vi "BoxcarAverage.vi"(2 "IR Sensors In":T1(array[cluster]), 3 "Box Car Average In":dbl[][](array[numeric])) -> (0 "IR Sensors Out":T1(array[cluster]), 1 "Box Car Average Out":dbl[][](array[numeric]))   [LabVIEW 2014]
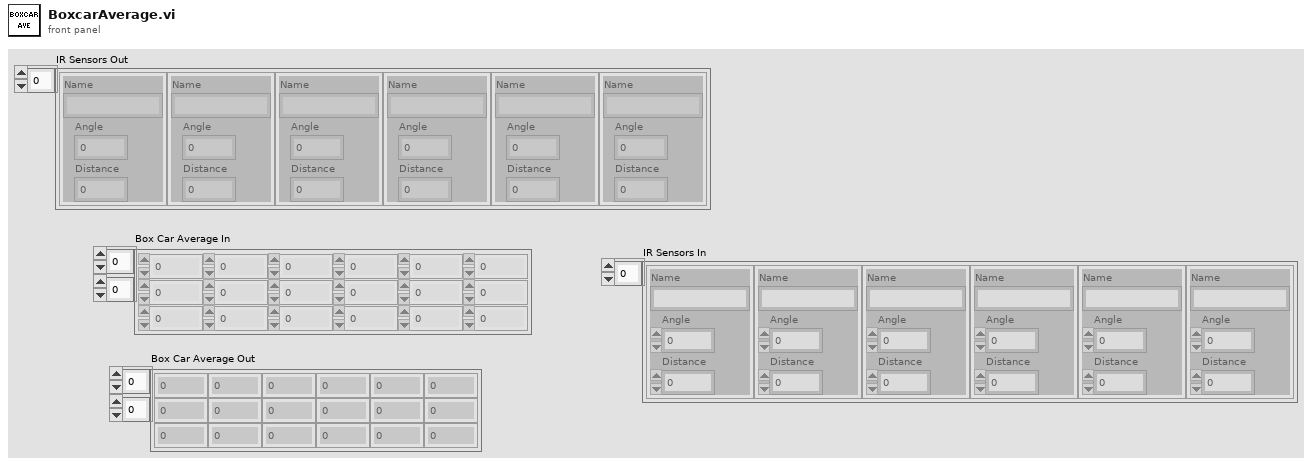
[diagram p1: front panel]
types:
  T1 = cluster{"Name":string, "Angle":dbl, "Distance":dbl}[]
  T2 = cluster{"Name":string, "Angle":dbl, "Distance":dbl}
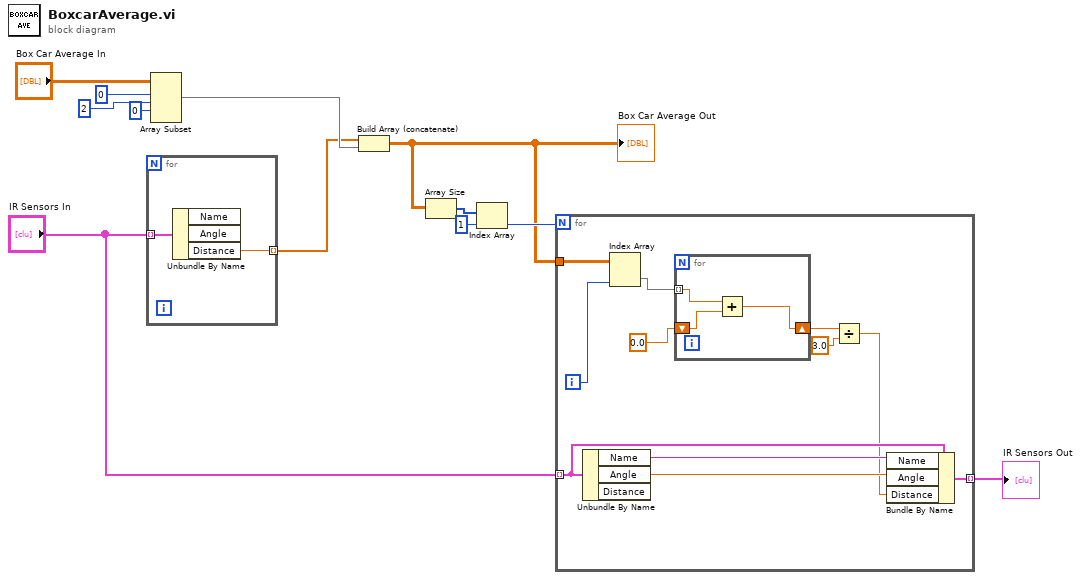
[diagram p0: block diagram]
diagram:
  n1 = for {
    tunnel: "IR Sensors In" -> [w14] mode=indexing
    tunnel: [w13] -> w7 mode=indexing
    n2 = Unbundle By Name(w14) -> ("Distance"=w13:dbl)  [unwired: 2 out]
  }
  n3 = Array Subset(array="Box Car Average In", index (row)=0 ("index"), length (row)=2 ("length"), index (col)=0 ("index")) -> (w8:dbl[][])  [unwired: 1 in]
  n4 = Build Array (concatenate)(w7, w8) -> (w3:dbl[][])
  "Box Car Average Out" <- w3
  n5 = Array Size(array=w3) -> (size(s)=w6:i32[])
  n6 = Index Array(array=w6, index=1) -> (element=w4:i32)
  n7 = for {
    N: w4 -> [_]
    tunnel: w3 -> [w25]
    tunnel: "IR Sensors In" -> [w19] mode=indexing
    tunnel: [w15] -> w1 mode=indexing
    i -> [w24]
    n8 = Unbundle By Name(w19) -> ("Name"=w18:string, "Angle"=w17:dbl)  [unwired: 1 out]
    n9 = Index Array(array=w25, index (col)=w24) -> (element=w23:dbl[])  [unwired: 1 in]
    n10 = for {
      tunnel: w23 -> [w28] mode=indexing
      shift-right: [w26] -> w21
      shift-left: 0.0 -> [w27]
      n11 = Add(x=w28, y=w27) -> (x+y=w26:dbl)
    }
    n12 = Divide(x=w21, y=3.0) -> (x/y=w16:dbl)
    n13 = Bundle By Name(cluster=w19, "Name"=w18, "Angle"=w17, "Distance"=w16) -> (w15:T2)
  }
  "IR Sensors Out" <- w1
